vi "Buffer Configure.vi"(5 "Collect Timestamps (Off)":bool, 6 "Timestamp Resolution (0.000001)":dbl=1e-06, 7 "Collect Source Values (Off)":bool, 8 "error in (no error)":errorcluster, 9 "Buffer Name":string, 10 "Append Mode (Off)":bool, 11 "VISA resource name":refnum<visa-resource-name>) -> (0 "error out":errorcluster, 3 "VISA resource name out":refnum<visa-resource-name>, 4 "Command String":string)   [LabVIEW 2012, in "Keithley 2600 Series.lvlib"]
doc: "This VI is used to configure the properties of a reading buffer. It is used to adjust the buffer's timestamp resolution and turn on or off append mode, collection of source value and collection of timestamps.\n\n<b>Note:</b> The reading buffer must be cleared before calling this VI else a TSP error will occur."
uses:
  Keithley 2600 Series.lvlib
  Private/GlobalVariables.vi
panel:
  # "(c) 2008 Keithley Instruments, Inc.  ALL RIGHTS RESERVED."
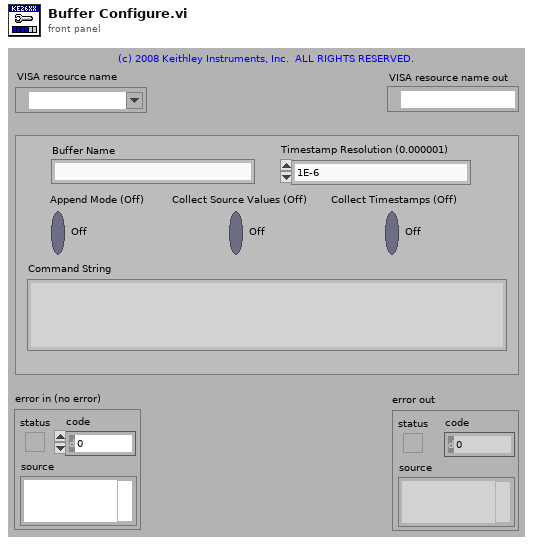
[diagram p1: front panel]
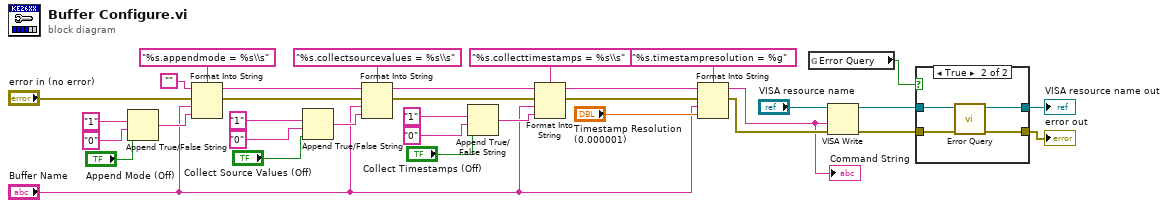
[diagram p0: block diagram]
diagram:
  n1 = Append True/False String(1:"Append Mode (Off)", 2:"0" ("false string"), 3:"1" ("true string")) -> (0:w8:string)  [unwired: 1 out]
  n2 = Format Into String(format string="%s.appendmode = %s\\s", initial string="", error in="error in (no error)", "Buffer Name", w8) -> (resulting string=w12:string, error out=w15:errorcluster)
  n3 = Append True/False String(1:"Collect Source Values (Off)", 2:"0" ("false string"), 3:"1" ("true string")) -> (0:w7:string)  [unwired: 1 out]
  n4 = Format Into String(format string="%s.collectsourcevalues = %s\\s", initial string=w12, error in=w15, "Buffer Name", w7) -> (resulting string=w11:string, error out=w14:errorcluster)
  n5 = Append True/False String(1:"Collect Timestamps (Off)", 2:"0" ("false string"), 3:"1" ("true string")) -> (0:w6:string)  [unwired: 1 out]
  n6 = Format Into String(format string="%s.collecttimestamps = %s\\s", initial string=w11, error in=w14, "Buffer Name", w6) -> (resulting string=w10:string, error out=w13:errorcluster)
  n7 = Format Into String(format string="%s.timestampresolution = %g", initial string=w10, error in=w13, "Buffer Name", "Timestamp Resolution (0.000001)") -> (resulting string=w1:string, error out=w2:errorcluster)
  "Command String" <- w1
  n8 = global read "GlobalVariables.vi" "Error Query"() -> (w25:bool)
  n9 = VISA Write(VISA resource name="VISA resource name", write buffer=w1, error in (no error)=w2) -> (VISA resource name out=w24:refnum<visa-resource-name>, error out=w23:errorcluster)  [unwired: 1 out]
  n10 = case shown="True" w25 {
    tunnel: w24 -> [w36 w40]
    tunnel: w23 -> [w35 w39]
    tunnel: [w36 w38] -> w21
    tunnel: [w35 w37] -> w22
    frame False {
    }
    frame True {
      n11 = call "Error Query.vi"("error in (no error)"=w39, "VISA resource name"=w40) -> ("error out"=w37:errorcluster, "VISA resource name out"=w38:refnum<visa-resource-name>)  [unwired: 8 out]
    }
  }
  "VISA resource name out" <- w21
  "error out" <- w22
